vi "NF LI56xx u_make command.vi"(9 "string format":string, 11 "input string":string) -> (3 "output string":string)   [LabVIEW 2019]
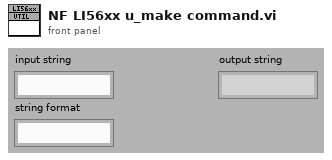
[diagram p1: front panel]
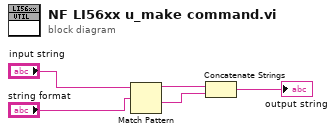
[diagram p0: block diagram]
diagram:
  n1 = Match Pattern(string="input string", regular expression="string format") -> (before substring=w3:string, after substring=w2:string)  [unwired: 1 in, 2 out]
  n2 = Concatenate Strings(w3, w2) -> (→"output string":string)
